vi "Shutdown.vi"(8 "error in":errorcluster, 11 "eCRDS in":refnum<class "eCRDS.lvclass">) -> (0 "error out":errorcluster, 3 "eCRDS out":refnum<class "eCRDS.lvclass">)   [LabVIEW 2014, in "eCRDS Library.lvlib" / "eCRDS.lvclass"]
uses:
  eCRDS.lvclass
  eCRDS.lvclass/eCRDS.ctl
  reusable/CRDS/Main/CRDS.lvclass
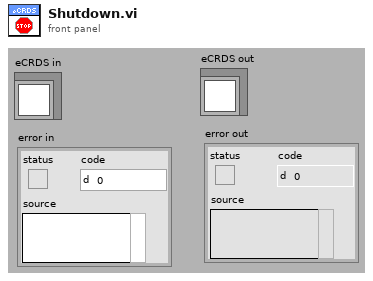
[diagram p1: front panel]
types:
  T1 = cluster{"CLk":refnum<k21>, "AI":refnum<k21>, "DO":refnum<k21>}
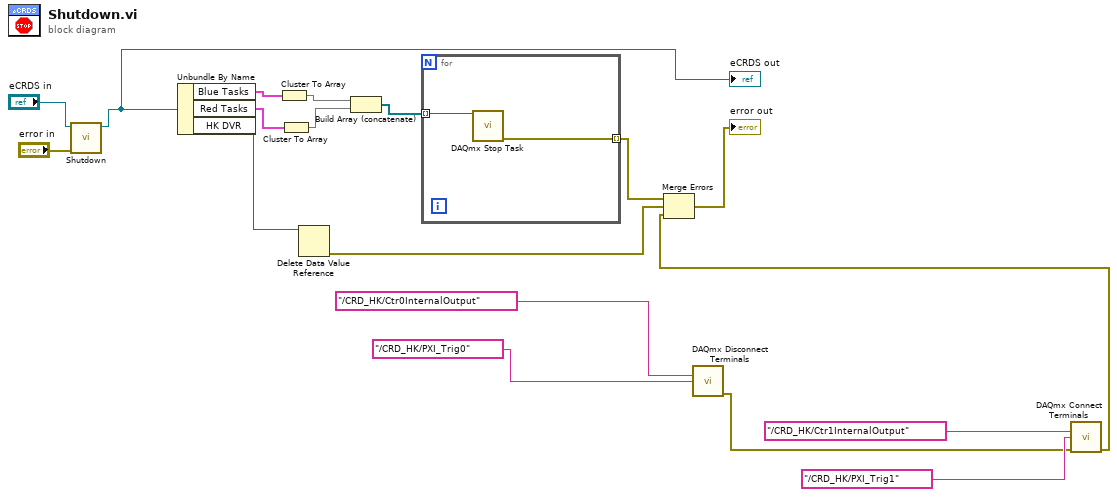
[diagram p0: block diagram]
diagram:
  n1 = call-parent "Shutdown.vi"("error in"="error in", "Instrument in"="eCRDS in") -> ("Instrument out"=w5:refnum<class "eCRDS.lvclass">)  [unwired: 8 in, 1 out]
  "eCRDS out" <- w5
  n2 = Unbundle By Name(w5) -> ("Blue Tasks"=w11:T1, "Red Tasks"=w9:T1, "HK DVR"=w4:refnum<data-value>)
  n3 = Cluster To Array(cluster=w11) -> (array=w10:refnum<k21>[])
  n4 = Cluster To Array(cluster=w9) -> (array=w8:refnum<k21>[])
  n5 = Delete Data Value Reference(data value reference=w4) -> (error out=w3:errorcluster)  [unwired: 1 in, 1 out]
  n6 = Build Array (concatenate)(w10, w8) -> (w7:refnum<k21>[])
  n7 = for {
    tunnel: w7 -> [w20] mode=indexing
    tunnel: [w19] -> w6 mode=indexing
    n8 = call <vilib>:"DAQmx Stop Task.vi"("task/channels in"=w20) -> ("error out"=w19:errorcluster)  [unwired: 13 in, 1 out]
  }
  n9 = call <vilib>:"DAQmx Disconnect Terminals.vi"("source terminal"=tag "/CRD_HK/Ctr0InternalOutput", "destination terminal"=tag "/CRD_HK/PXI_Trig0") -> ("error out"=w12:errorcluster)  [unwired: 13 in]
  n10 = call <vilib>:"DAQmx Connect Terminals.vi"("source terminal"=tag "/CRD_HK/Ctr1InternalOutput", "destination terminal"=tag "/CRD_HK/PXI_Trig1", "error in"=w12) -> ("error out"=w2:errorcluster)  [unwired: 12 in]
  n11 = Merge Errors(w6, w3, w2) -> (→"error out":errorcluster)
